vi "Get All Status.vi"(8 "error in (no error)":errorcluster, 11 "Instrument Ref In":refnum<k24>) -> (0 "error out":errorcluster, 1 "Field\nStatus":i32(ring) items=["MagnetUnknown"=0, "StablePersistent"=1, "WarmingSwitch"=2, "CoolingSwitch"=3, "StableDriven"=4, "Iterating"=5, "Charging"=6, "Discharging"=7, "CurrentError"=8, "MagnetFailure"=15], 2 "Temperature\nStatus":i32(ring) items=["TemperatureUnknown"=0, "Stable"=1, "Tracking"=2, "Near"=5, "Chasing"=6, "Filling"=7, "Standby"=10, "Disabled"=13, "ImpedanceNotFunction"=14, "TempFailure"=15], 3 "Instrument Ref Out":refnum<k24>, 4 "Field":dbl, 5 "Chamber\nStatus":i32(ring) items=["ChamberUnknown"=0, "PurgedAndSealed"=1, "VentedAndSealed"=2, "Sealed"=3, "Purging"=4, "Venting"=5, "PreHiVac"=6, "HighVac"=7, "PumpContinuous"=8, "VentContinuous"=9, "ChamberFailure"=15], 6 "Temperature":dbl, 7 "Position":dbl)   [LabVIEW 2020]
uses:
  C:/Users/QDUser/Desktop/LabVIEW Programs/PPMS Interface/dev/QDInstrument/QDInstrument.dll
  dev/QDInstrument/QDInstrument.dll
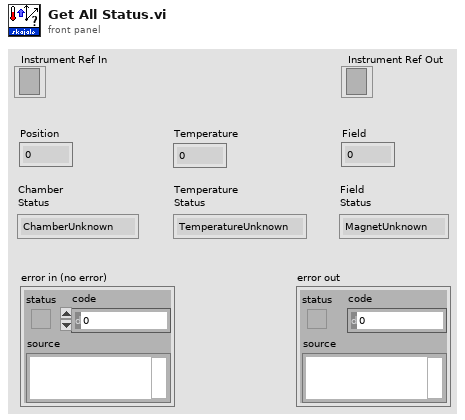
[diagram p1: front panel]
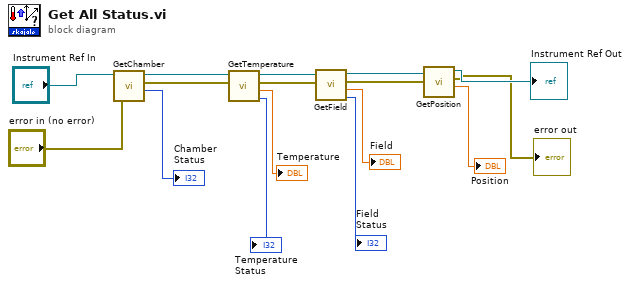
[diagram p0: block diagram]
diagram:
  n1 = call "GetChamber.vi"("error in (no error)"="error in (no error)", "Instrument Ref In"="Instrument Ref In") -> ("Chamber\nStatus"=→"Chamber\nStatus":i32, "error out"=w7:errorcluster, "Instrument Ref Out"=w12:refnum<k24>)  [unwired: 2 in, 1 out]
  n2 = call "GetTemperature.vi"("error in (no error)"=w7, "Instrument Ref In"=w12) -> ("Temperature\nStatus"=→"Temperature\nStatus":i32, "Temperature"=→"Temperature":dbl, "error out"=w6:errorcluster, "Instrument Ref Out"=w11:refnum<k24>)  [unwired: 3 in, 1 out]
  n3 = call "GetField.vi"("error in (no error)"=w6, "Instrument Ref In"=w11) -> ("Field\nStatus"=→"Field\nStatus":i32, "Field"=→"Field":dbl, "error out"=w5:errorcluster, "Instrument Ref Out"=w4:refnum<k24>)  [unwired: 3 in, 1 out]
  n4 = call "GetPosition.vi"("error in (no error)"=w5, "Instrument Ref In"=w4) -> ("Position"=→"Position":dbl, "error out"=→"error out":errorcluster, "Instrument Ref Out"=→"Instrument Ref Out":refnum<k24>)  [unwired: 2 in, 1 out]
